vi "Trajectory_selection.vi"(8 "Matrices":T2, 9 "Configuration":T1={"Accelerometer Bias"={"X (m/s)"=0.0, "Y (m/s)"=0.0, "Z (m/s)"=0.0}, "Gyroscope Bias"={"X (m/s)"=0.0, "Y (m/s)"=0.0, "Z (m/s)"=0.0}, "Steering Motor Gear Ratio"=611.0, "Steering Pully Gear Ratio"=1.0, "Steering Encoder CPR"=500.0, "Steering Motor Max RPM"=4000.0, "Wheelbase (m)"=1.12, "Fork Angle (rad)"=1.3, "Balancing Controller"={"Kp (/s)"=1.0, "Kd (1)"=1.0}, "Max Allowed Steering Angle (rad)"=0.7, "Task Periods"={"Emergency Stop (us)"=10000, "IMU (us)"=10000, "Steering Motor Encoder (us)"=10000, "State Estimator (us)"=10000, "Balancing Controller (us)"=10000, "GNSS (us)"=10000, "Logging (us)"=50000, "Drive Motor (us)"=100000, "Visualization (us)"=100000}, "Drive Motor Gear Ratio"=0.7, "lr"=0.0, "lf"=0.0, "lambda"=0.0, "k1"=0.0, "k2"=0.0, "e1_max"=0.0, "Ad_t"=0.0, "Bd_t"=0.0, "C_t"=0.0, "D_t"=0.0, "Wheel radius"=0.311}) -> (0 "RefTraj out":refnum<data-value>)   [LabVIEW 2021]
uses:
  Configuration/Configuration.ctl
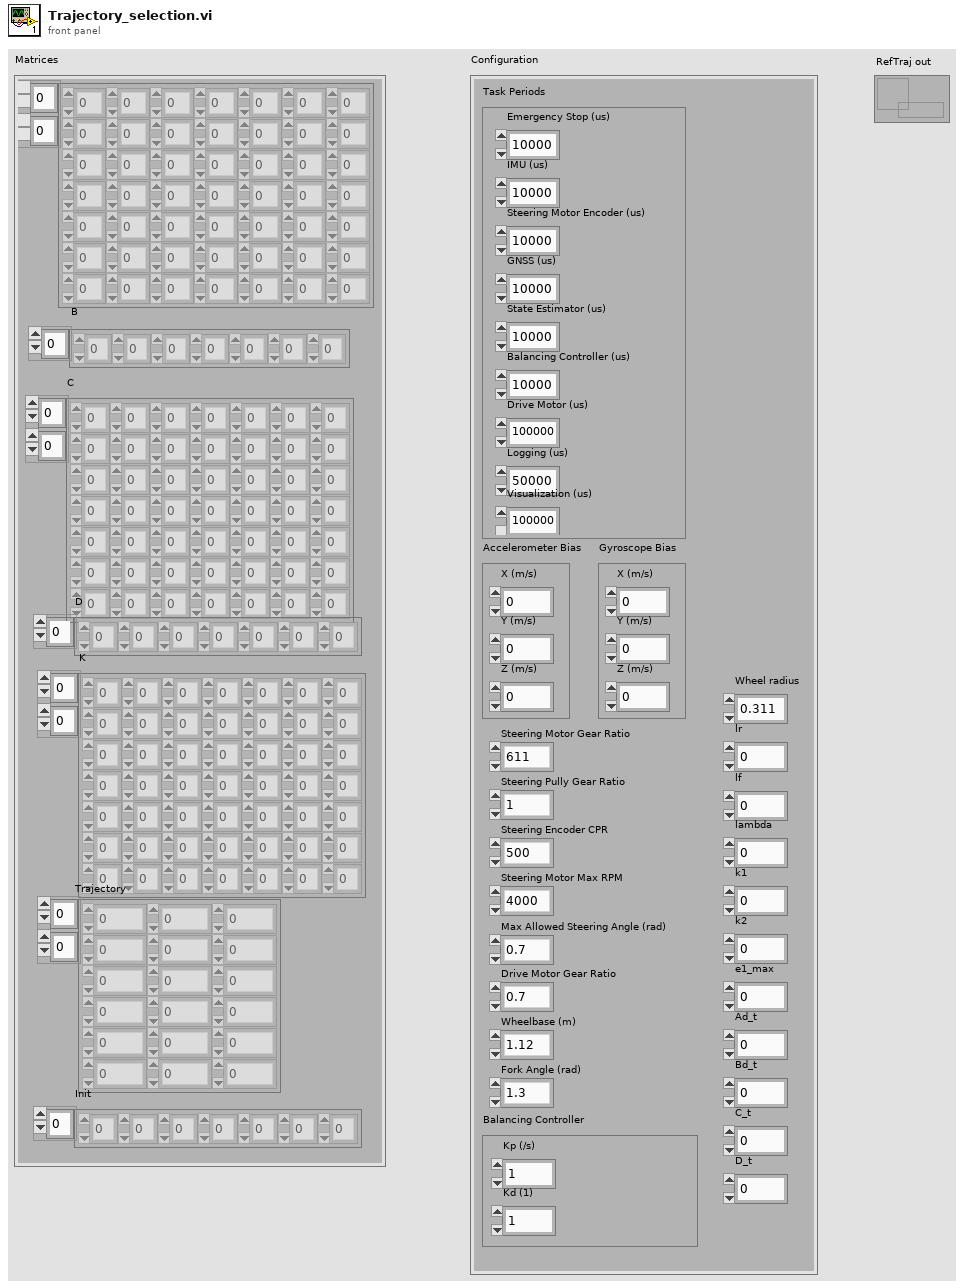
[diagram p1: front panel]
types:
  T1 = typedef "Configuration.ctl" = cluster{"Accelerometer Bias":cluster{"X (m/s)":dbl, "Y (m/s)":dbl, "Z (m/s)":dbl}, "Gyroscope Bias":cluster{"X (m/s)":dbl, "Y (m/s)":dbl, "Z (m/s)":dbl}, "Steering Motor Gear Ratio":dbl, "Steering Pully Gear Ratio":dbl, "Steering Encoder CPR":dbl, "Steering Motor Max RPM":dbl, "Wheelbase (m)":dbl, "Fork Angle (rad)":dbl, "Balancing Controller":cluster{"Kp (/s)":dbl, "Kd (1)":dbl}, "Max Allowed Steering Angle (rad)":dbl, "Task Periods":cluster{"Emergency Stop (us)":i64, "IMU (us)":i64, "Steering Motor Encoder (us)":i64, "State Estimator (us)":i64, "Balancing Controller (us)":i64, "GNSS (us)":i64, "Logging (us)":i64, "Drive Motor (us)":i64, "Visualization (us)":i64}, "Drive Motor Gear Ratio":dbl, "lr":dbl, "lf":dbl, "lambda":dbl, "k1":dbl, "k2":dbl, "e1_max":dbl, "Ad_t":dbl, "Bd_t":dbl, "C_t":dbl, "D_t":dbl, "Wheel radius":dbl}
  T2 = cluster{"B":dbl[], "A":dbl[][], "C":dbl[][], "D":dbl[], "K":dbl[][], "Trajectory":dbl[][], "Init":dbl[]}
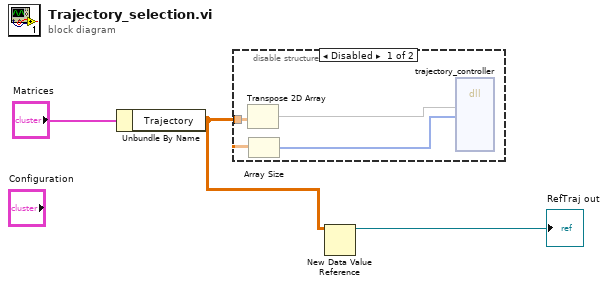
[diagram p0: block diagram]
diagram:
  n1 = Unbundle By Name("Matrices") -> ("Trajectory"=w2:dbl[][])
  n2 = disable-structure shown="Disabled" {
    disable-tunnel: w2 -> [w4 _]
    frame Disabled {
      n3 = Transpose 2D Array(2D array=w4) -> (transposed array=w6:dbl[][])
      n4 = Array Size(array=w4) -> (size(s)=w5:i32[])
      n5 = dll-call lib="libtrajectory_controller.so" fn="trajectory_controller"("Traj"=w6, "traj_size"=w5) -> ()  [unwired: 14 in, 2 out]
    }
    frame Enabled {
    }
  }
  n6 = New Data Value Reference(data value=w2) -> (data value reference=→"RefTraj out":refnum<data-value>)  [unwired: 1 in, 1 out]
